vi "Collect additional metadata.vi"(8 "error in (no error)":errorcluster, 10 "hours":dbl, 11 "Data Fields":T1) -> (0 "error out":errorcluster, 2 "Error":bool, 3 "appended array":string[][](array[string]))   [LabVIEW 2013]
uses:
  <vilib>/Utility/file.llb/Read From Spreadsheet File (string).vi
  <vilib>/Utility/file.llb/Write To Spreadsheet File (string).vi
panel:
  out "data string":string
  # "ambient temp (sphere)"
  # "ambient temp room"
  # "Fill out the follow data fields for each test. An error will be thrown if any data fields are missing.\nNew parameters for data fields can be added by right clicking, hitting \"properties\", then \"edit items\""
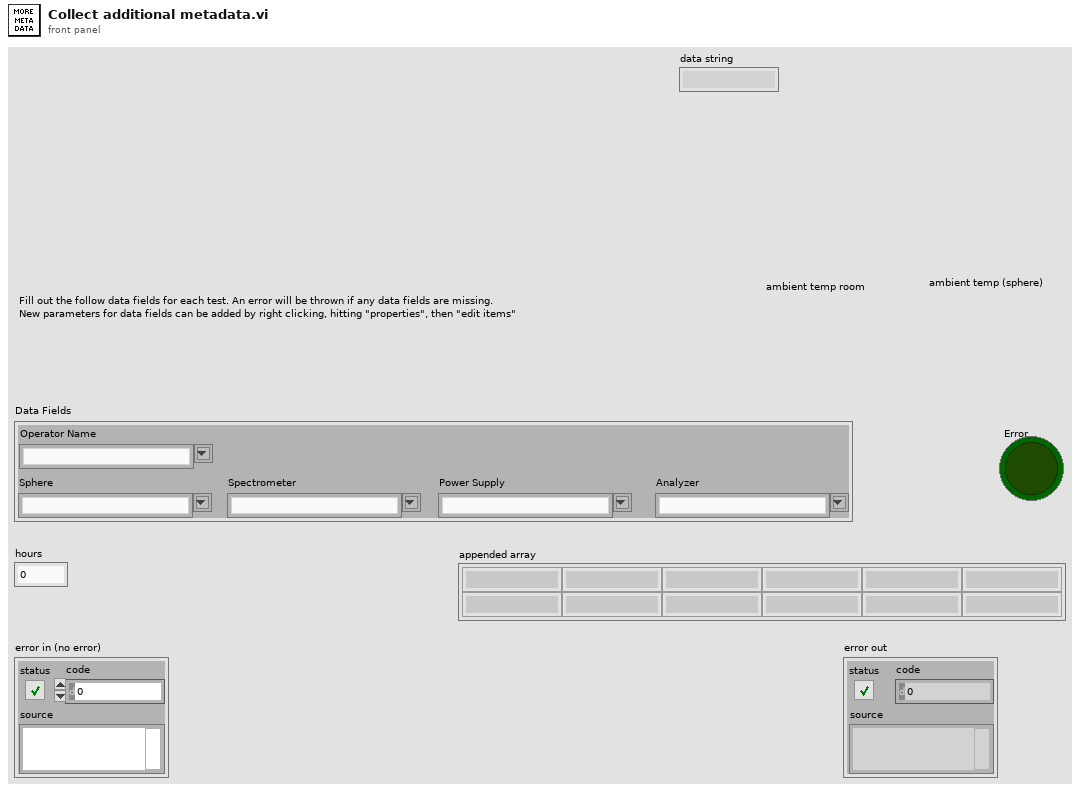
[diagram p1: front panel]
types:
  T1 = cluster{"Sphere":string, "Spectrometer":string, "Power Supply":string, "Analyzer":string, "Operator Name":string}
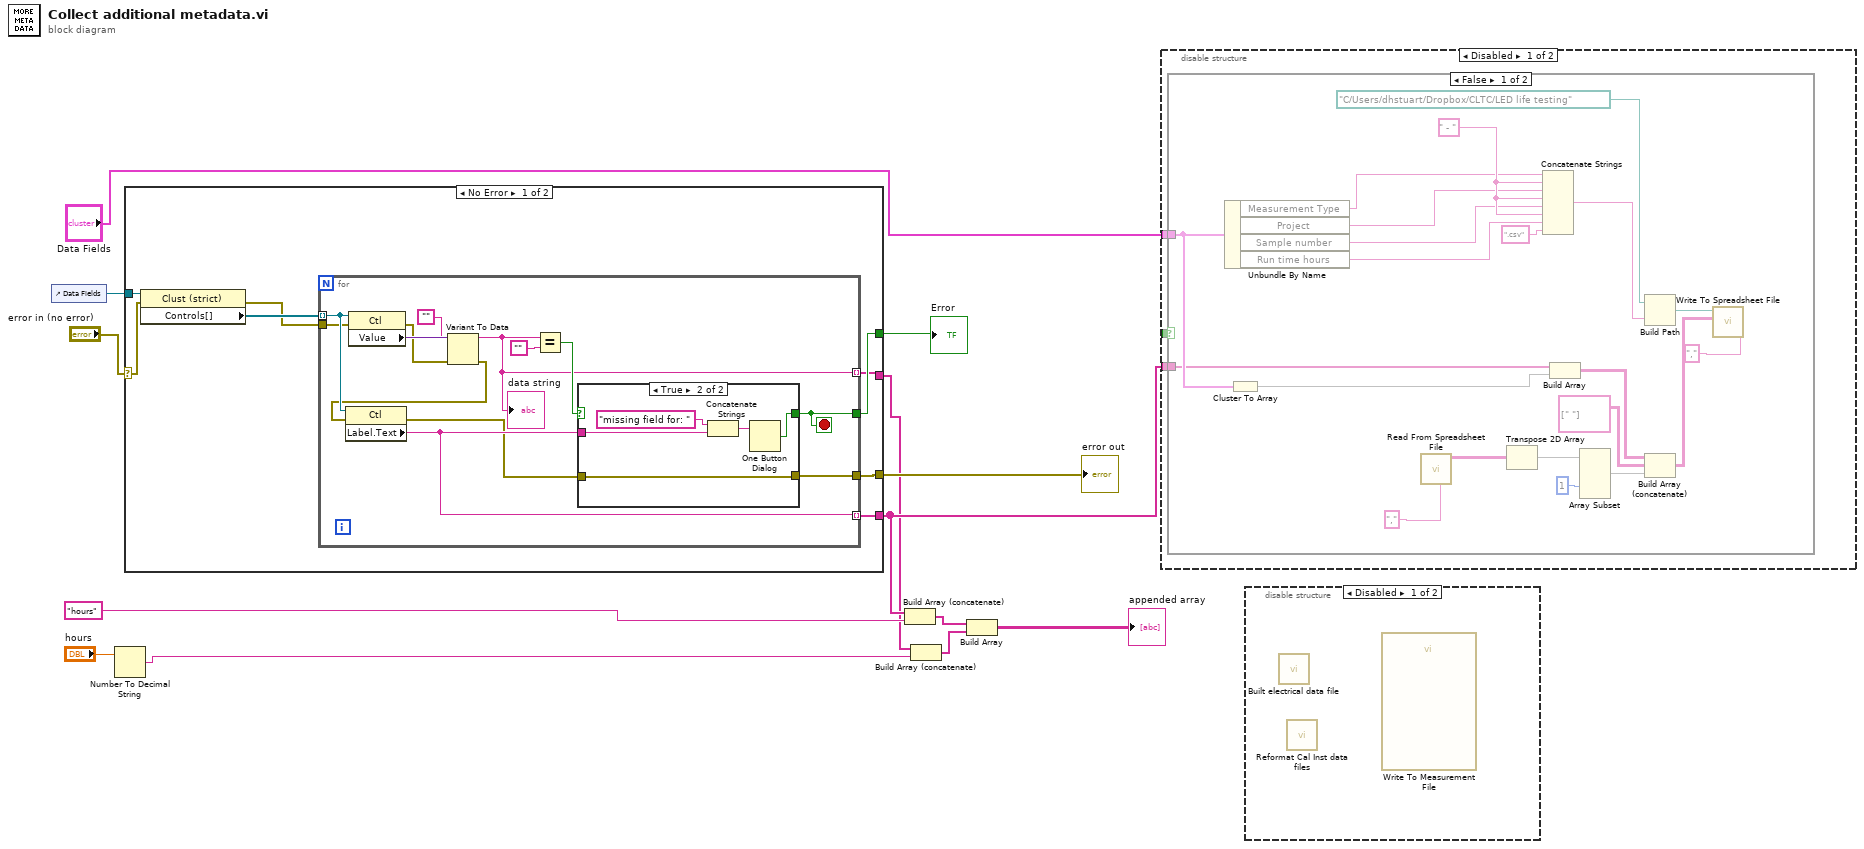
[diagram p0: block diagram]
diagram:
  n1 = control-ref of="Data Fields"() -> (w13:refnum<vi>)
  n2 = Number To Decimal String(number="hours") -> (decimal integer string=w4:string)  [unwired: 1 in]
  n3 = case shown="No Error" "error in (no error)" {
    selector: "error in (no error)" -> [w16 w42]
    tunnel: w13 -> [w21 _]
    tunnel: [w19 _] -> w12
    tunnel: [w18 _] -> w6
    tunnel: [w15 w42] -> w9
    tunnel: [w14 _] -> w3
    frame No Error {
      n4 = property class="Clust (strict)"(reference=w21, error in=w16) -> (error out=w17:errorcluster, "Controls[]"=w20:refnum<vi>[])  [unwired: 1 out]
      n5 = for {
        tunnel: w20 -> [w31] mode=indexing
        tunnel: [w34] -> w19
        tunnel: [w28] -> w18 mode=indexing
        tunnel: w17 -> [w27]
        tunnel: [w23] -> w15
        tunnel: [w22] -> w14 mode=indexing
        stop <- w34 stop-if-true
        n6 = property class="Ctl"(reference=w31, error in=w27) -> (error out=w26:errorcluster, "Value"=w32:variant)  [unwired: 1 out]
        n7 = Variant To Data(error in=w26, type="", Variant=w32) -> (data=w22:string, error out=w25:errorcluster)
        "data string" <- w22
        n8 = property class="Ctl"(reference=w31, error in=w25) -> (error out=w24:errorcluster, "Label.Text"=w28:string)  [unwired: 1 out]
        n9 = Equal?(x=w22, y="") -> (x = y?=w33:bool)
        n10 = case shown="True" w33 {
          selector: w33 -> [w36 _]
          tunnel: w28 -> [_ w40]
          tunnel: [w36 w38] -> w34
          tunnel: w24 -> [w35 w37]
          tunnel: [w35 w37] -> w23
          frame False {
          }
          frame True {
            n11 = Concatenate Strings("missing field for: ", w40) -> (w39:string)
            n12 = One Button Dialog(message=w39) -> (true=w38:bool)  [unwired: 1 in]
          }
        }
      }
    }
    frame Error {
    }
  }
  "error out" <- w9
  "Error" <- w12
  n13 = Build Array (concatenate)(w6, "hours") -> (w1:string[])
  n14 = Build Array (concatenate)(w3, w4) -> (w2:string[])
  n15 = Build Array(w1, w2) -> (→"appended array":string[][])
  n16 = disable-structure shown="Disabled" {
    disable-tunnel: _ -> [w45 _]
    disable-tunnel: "Data Fields" -> [w44 _]
    disable-tunnel: w6 -> [w43 _]
    frame Disabled {
      n17 = case shown="False" w45 {
        tunnel: w44 -> [w52 _]
        tunnel: w43 -> [w51 _]
        frame False {
          w66 = " - "
          n18 = Unbundle By Name(w52) -> ("Measurement Type"=w49:string, "Project"=w48:string, "Sample number"=w47:string, "Run time hours"=w46:string)
          n19 = Cluster To Array(cluster=w52) -> (array=w50:string[])
          n20 = call-poly <vilib>:"Read From Spreadsheet File.vi"("delimiter (\\t)"="," ("delimiter (\\t)")) -> ("all rows"=w63:string[][])  [unwired: 6 in, 4 out]
          n21 = Transpose 2D Array(2D array=w63) -> (transposed array=w58:string[][])
          n22 = Concatenate Strings(w49, w66, w48, w66, w47, w66, w46, ".csv" ("string")) -> (w54:string)
          n23 = Build Array(w51, w50) -> (w64:string[][])
          n24 = Array Subset(array=w58, index (col)=1 ("index")) -> (w57:string[][])  [unwired: 3 in]
          n25 = Build Path(base path=path "C:/Users/dhstuart/Dropbox/CLTC/LED life testing" ("file path (dialog if empty)"), name or relative path=w54) -> (appended path=w53:path)
          n26 = Build Array (concatenate)(w64, string[][] [[" "]] ("array"), w57) -> (w61:string[][])
          n27 = call-poly <vilib>:"Write To Spreadsheet File.vi"("delimiter (\\t)"="," ("delimiter (\\t)"), "2D data"=w61, "file path (dialog if empty)"=w53) -> ()  [unwired: 5 in, 1 out]
        }
        frame True {
        }
      }
    }
    frame Enabled {
    }
  }
  n28 = disable-structure shown="Disabled" {
    frame Disabled {
      n29 = call "Built electrical data file.vi"() -> ()  [unwired: 11 in, 1 out]
      n30 = call "Reformat Cal Inst data files.vi"() -> ()  [unwired: 11 in, 1 out]
      n31 = call "Write To Measurement File"() -> ()  [unwired: 17 in, 3 out]
    }
    frame Enabled {
    }
  }
